vi "LSX Set Stop Accel.vi"(6 "dAD":dbl, 7 "dZD":dbl, 8 "error in (no error)":errorcluster, 9 "dYD":dbl, 10 "dXD":dbl, 11 "lLSID":i32) -> (0 "error out":errorcluster, 3 "function return":i32)   [LabVIEW 2016, in "Tango_DLL.lvlib"]
doc: "TANGOAPI int TANGOCALL LSX_SetStopAccel (int lLSID, double dXD, double dYD, double dZD, double dAD);"
uses:
  Tango_DLL.lvlib
  2017/Microscope Control/Device Library/Stages/Marzhauser/SCAN IM 120 x 80/Tango DLL VIs/Tango_DLL.dll
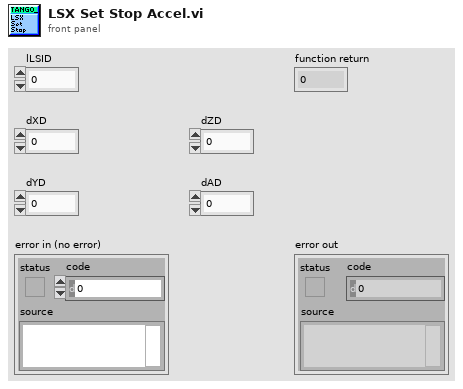
[diagram p1: front panel]
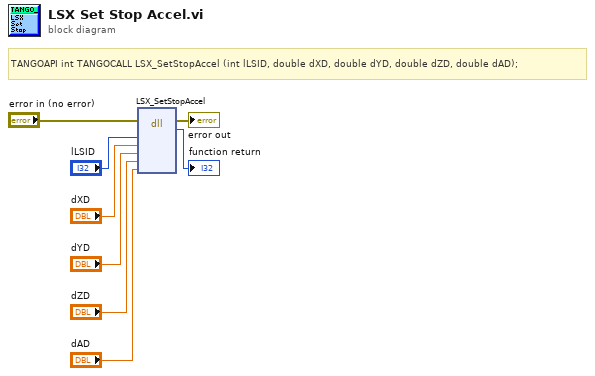
[diagram p0: block diagram]
diagram:
  # "TANGOAPI int TANGOCALL LSX_SetStopAccel (int lLSID, double dXD, double dYD, double dZD, double dAD);"
  n1 = dll-call lib="C:/Users/4PiSMS/Documents/Microscope Control/2017/Microscope Control/Device Library/Stages/Marzhauser/SCAN IM 120 x 80/Tango DLL VIs/Tango_DLL.*" fn="LSX_SetStopAccel"(error in="error in (no error)", "lLSID"="lLSID", "dXD"="dXD", "dYD"="dYD", "dZD"="dZD", "dAD"="dAD") -> (error out=→"error out":errorcluster, →"function return":i32)  [unwired: 7 in, 1 out]
